vi "Read.vi"(11 "Test Case In":refnum<class "Test PCANBasic.lvclass">) -> (0 "error out":errorcluster, 3 "Test Case Out":refnum<class "Test PCANBasic.lvclass">)   [LabVIEW 2025, in "Test PCANBasic.lvclass"]
uses:
  Test PCANBasic.lvclass
  C:/Program Files/National Instruments/LabVIEW 2025/vi.lib/Astemes/LUnit/Test Case.lvclass
  source/PCAN Message.ctl
  source/PCAN Message types.ctl
  source/PCAN Baud.ctl
  source/TPCANHandle.ctl
  <vilib>/Astemes/LUnit/Test Case.lvclass/Test Case.ctl
  <vilib>/Astemes/LUnit/Core/LUnit Test Case/Private/Append Pass Result.vi
  <vilib>/Astemes/LUnit/Core/LUnit Test Case/Private/Append Fail Result.vi
  <vilib>/Astemes/LUnit/Core/LUnit Test Case/Private/Run In UI.vi
  <vilib>/Utility/error.llb/Clear Errors.vi
  Test PCANBasic.lvclass/Test PCANBasic.ctl
  source/PCANBasic.lvlib
  <vilib>/Astemes/LUnit/Test Case.lvclass
panel:
  out "PCAN Message":T1 {"DATA"."7" format="%.0x"; "DATA"."6" format="%.0x"; "DATA"."5" format="%.0x"; "DATA"."4" format="%.0x"; "DATA"."3" format="%.0x"; "DATA"."2" format="%.0x"; "DATA"."1" format="%.0x"; "MSGTYPE" items=["STANDARD"=0, "RTR"=1, "EXTENDED"=2, "FD"=4, "BRS"=8, "ESI"=16, "ECHO"=32, "ERRFRAME"=64, "STATUS"=128]}
  out "Time Stamp":timestamp format="%<%x %.3X>T"
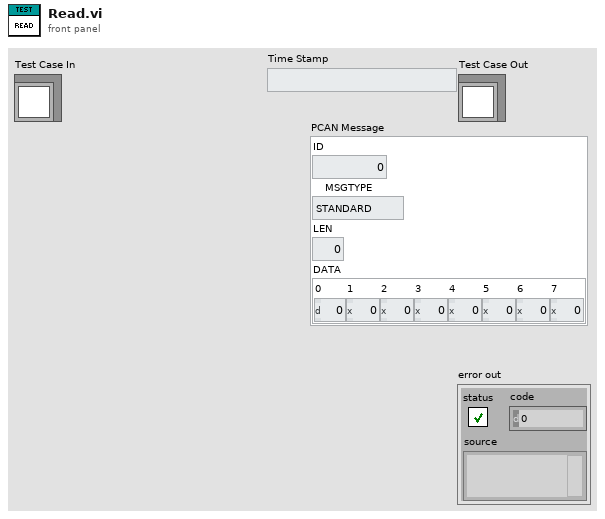
[diagram p1: front panel]
types:
  T1 = typedef "PCANBasic.lvlib/PCAN Message.ctl" = cluster{"ID":u32, "MSGTYPE":T2, "LEN":u8, "DATA":cluster{"0":u8, "1":u8, "2":u8, "3":u8, "4":u8, "5":u8, "6":u8, "7":u8}}
  T2 = typedef "PCANBasic.lvlib/PCAN Message types.ctl" = u8
  T3 = typedef "PCANBasic.lvlib/TPCANHandle.ctl" = u16
  T4 = typedef "PCANBasic.lvlib/PCAN Baud.ctl" = u16
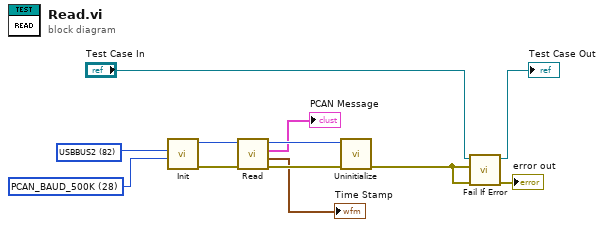
[diagram p0: block diagram]
diagram:
  w8 = T3 82 items=["USBBUS1"=81, "USBBUS2"=82, "USBBUS3"=83, "USBBUS4"=84, "USBBUS5"=85, "USBBUS6"=86, "USBBUS7"=87, "USBBUS8"=88, "USBBUS9"=1289, "USBBUS10"=1290, "USBBUS11"=1291, "USBBUS12"=1292, "USBBUS13"=1293, "USBBUS14"=1294, "USBBUS15"=1295, "USBBUS16"=1296] ("Channel")
  w9 = T4 28 items=["PCAN_BAUD_1M"=20, "PCAN_BAUD_800K"=22, "PCAN_BAUD_500K"=28, "PCAN_BAUD_250K"=284, "PCAN_BAUD_125K"=796, "PCAN_BAUD_100K"=17199, "PCAN_BAUD_95K"=49998, "PCAN_BAUD_83K"=34091, "PCAN_BAUD_50K"=18223, "PCAN_BAUD_47K"=5140, "PCAN_BAUD_33K"=35631, "PCAN_BAUD_20K"=21295, "PCAN_BAUD_10K"=26415, "PCAN_BAUD_5K"=32639] ("Baudrate")
  n1 = call "Init.vi"("Baudrate"=w9, "Channel"=w8) -> ("error out"=w7:errorcluster, "TPCANHandle"=w5:T3)  [unwired: 7 in, 1 out]
  n2 = call "Read.vi"("error in"=w7, "TPCANHandle"=w5) -> ("error out"=w6:errorcluster, "Time Stamp"=→"Time Stamp":timestamp, "PCAN Message"=→"PCAN Message":T1, "TPCANHandle"=w4:T3)  [unwired: 4 in, 2 out]
  n3 = call "Uninitialize.vi"("error in"=w6, "TPCANHandle"=w4) -> ("error out"=w1:errorcluster)  [unwired: 8 in, 1 out]
  n4 = call <vilib>:"Fail If Error.vi"("error in (no error)"=w1, "Assert error"=w1, "LUnit Test Case In"="Test Case In") -> ("error out"=→"error out":errorcluster, "LUnit Test Case Out"=→"Test Case Out":refnum<class "Test PCANBasic.lvclass">)  [unwired: 7 in]
